vi "Periodic Tasks.vi"(8 "error in":errorcluster) -> ()   [LabVIEW 2012]
doc: "This VI runs in parallel to other tasks. It can contain as many user-defined periodic loops as you need. These can carry out PID or other sorts of timed response."
uses:
  <vilib>/Rock Robotics/WPI/Relay/WPI_RelayValue.ctl
  <vilib>/Rock Robotics/SystemInterfaces/Utilities/FPGA_UtilitiesLED Source.ctl
  <vilib>/Rock Robotics/SystemInterfaces/Utilities/FPGA_UtilitiesLED State.ctl
  Robot Global Data.vi
  <vilib>/Rock Robotics/WPI/Joystick/WPI_JoystickGetSetRefNum.vi
  <vilib>/Rock Robotics/WPI/RobotDrive/WPI_RobotDriveGetSetRefNum.vi
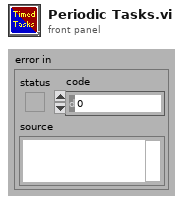
[diagram p1: front panel]
types:
  T1 = typedef "WPI_CompressorDevRef.ctl" = cluster{"DevStatus":errorcluster, "DigitalInputDevRef":T2, "RelayDevRef":T5}
  T2 = typedef "WPI_DigitalInputDevRef.ctl" = cluster{"DevStatus":errorcluster, "DIO Channel":T3, "Digital Module":T4}
  T3 = typedef "FPGA_DIOChannel.ctl" = enum8{"DIO 1", "DIO 2", "DIO 3", "DIO 4", "DIO 5", "DIO 6", "DIO 7", "DIO 8", "DIO 9", "DIO 10", "DIO 11", "DIO 12", "DIO 13", "DIO 14", "Invalid"}
  T4 = typedef "FPGA_TypedefDigitalModule.ctl" = enum16{"Digital Module 1", "Digital Module 2"}
  T5 = typedef "WPI_RelayDevRef.ctl" = cluster{"DevStatus":errorcluster, "Relay Channel":T6, "Digital Module":T4, "Relay Direction":T7}
  T6 = typedef "FPGA_DIORelayChannel.ctl" = enum8{"Relay 1", "Relay 2", "Relay 3", "Relay 4", "Relay 5", "Relay 6", "Relay 7", "Relay 8", "Invalid"}
  T7 = typedef "WPI_RelayDirection.ctl" = enum16{"Both directions", "Forward only", "Reverse only"}
  T8 = typedef "FPGA_UtilitiesLED State.ctl" = enum16{"Off", "On", "Toggle"}
  T9 = typedef "FPGA_UtilitiesLED Source.ctl" = enum16{"User LED", "FPGA LED"}
  T10 = typedef "WPI_RobotDriveDevRef.ctl" = cluster{"DevStatus":errorcluster, "Motors[]":T11[], "Square Inputs":bool, "Max Output":dbl, "Isochronous":bool}
  T11 = typedef "WPI_MotorControlDeviceRef.ctl" = cluster{"DeviceStatus":errorcluster, "Type":enum16{"PWM", "CAN"}, "PWM":cluster{"Digital Module":T4, "PWM Channel":T12, "DeadBand":T13}, "CAN":cluster{"Device Number":u8, "Control Mode":T14, "Semaphore":T15, "Max Vout":dbl}, "Invert":bool, "TransformRef":T16, "InvTransformRef":T16}
  T12 = typedef "FPGA_DIOPWMChannel.ctl" = enum8{"PWM 1", "PWM 2", "PWM 3", "PWM 4", "PWM 5", "PWM 6", "PWM 7", "PWM 8", "PWM 9", "PWM 10", "Invalid"}
  T13 = typedef "WPI_PWMDeadband.ctl" = cluster{"Name":string, "maxPositivePwm":i32, "minPositivePwm":i32, "centerPwm":i32, "maxNegativePwm":i32, "minNegativePwm":i32, "angularRange":u16}
  T14 = typedef "WPI_CANJaguar_ControlMode.ctl" = enum8{"Percent VBus", "Current", "Speed", "Position", "Voltage"}
  T15 = typedef "Semaphore RefNum" = refnum<k1>
  T16 = typedef "WPI_PWMTransform_ConPane.ctl" = refnum<vi>
  T17 = typedef "WPI_JoystickDevRef.ctl" = cluster{"Device":T18}
  T18 = typedef "WPI_JoystickDeviceEnum.ctl" = enum16{"USB 1", "USB 2", "USB 3", "USB 4", "Kinect 1", "Kinect 2"}
  T19 = cluster{"JoystickDevRef":T17, "RobotDriveDevRef":T10}
  T20 = typedef "WPI_RelayValue.ctl" = enum16{"Off", "On", "Forward", "Reverse"}
  T21 = typedef "WPI_JoystickButtonState.ctl" = cluster{"Button 1":bool, "Button 2":bool, "Button 3":bool, "Button 4":bool, "Button 5":bool, "Button 6":bool, "Button 7":bool, "Button 8":bool, "Button 9":bool, "Button 10":bool, "Button 11":bool, "Button 12":bool}
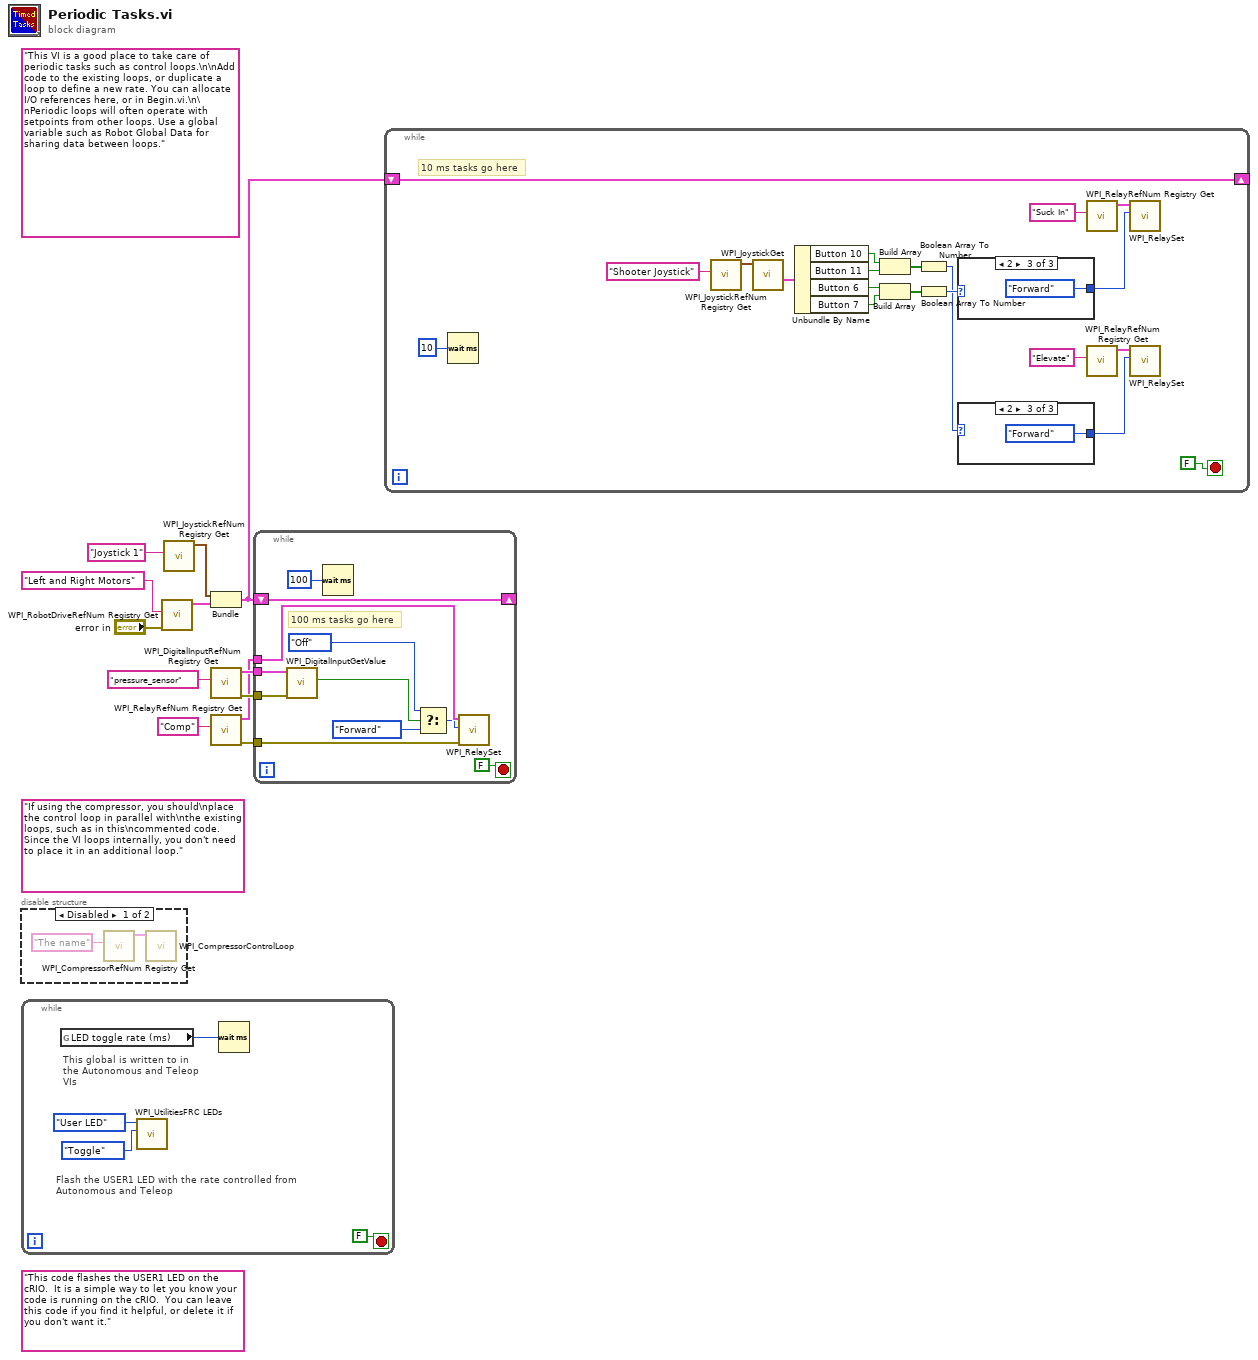
[diagram p0: block diagram]
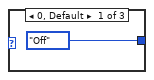
[diagram p3: hidden frame]
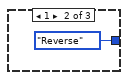
[diagram p4: hidden frame]
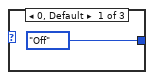
[diagram p5: hidden frame]
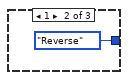
[diagram p6: hidden frame]
diagram:
  (unwired) "If using the compressor, you should\nplace the control loop in parallel with\nthe existing loops, such as in this\ncommented code. Since the VI loops internally, you don't need to place it in an additional loop."
  (unwired) "This code flashes the USER1 LED on the cRIO.  It is a simple way to let you know your code is running on the cRIO.  You can leave this code if you find it helpful, or delete it if you don't want it."
  (unwired) "This VI is a good place to take care of periodic tasks such as control loops.\n\nAdd code to the existing loops, or duplicate a loop to define a new rate. You can allocate I/O references here, or in Begin.vi.\n\nPeriodic loops will often operate with setpoints from other loops. Use a global variable such as Robot Global Data for sharing data between loops."
  n1 = disable-structure shown="Disabled" {
    frame Disabled {
      n2 = call <vilib>:"WPI_CompressorRefNum Registry Get.vi"("refnum name"="The name") -> ("CompressorDevRef"=w14:T1)  [unwired: 9 in, 1 out]
      n3 = call <vilib>:"WPI_CompressorControlLoop.vi"("CompressorDevRef"=w14) -> ()  [unwired: 11 in]
    }
    frame Enabled {
    }
  }
  n4 = while {
    stop <- FALSE stop-if-true
    # "This global is written to in the Autonomous and Teleop VIs"
    # "Flash the USER1 LED with the rate controlled from Autonomous and Teleop"
    n5 = global read "Robot Global Data.vi" "LED toggle rate (ms)"() -> (w15:u32)
    n6 = call <vilib>:"WPI_UtilitiesFRC LEDs.vi"("State"=FPGA_UtilitiesLED_State."Toggle", "LED Type"=FPGA_UtilitiesLED_Source."User LED") -> ()  [unwired: 1 in, 9 out]
    n7 = Wait (ms)(milliseconds to wait=w15) -> ()  [unwired: 1 out]
  }
  n8 = call <vilib>:"WPI_RobotDriveRefNum Registry Get.vi"("error in (no error)"="error in", "refnum name"="Left and Right Motors") -> ("RobotDriveDevRef"=w9:T10)  [unwired: 9 out]
  n9 = call <vilib>:"WPI_JoystickRefNum Registry Get.vi"("refnum name"="Joystick 1") -> ("JoystickDevRef"=w10:T17)  [unwired: 1 in, 9 out]
  n10 = Bundle("JoystickDevRef"=w10, "RobotDriveDevRef"=w9) -> (w8:T19)  [unwired: 1 out]
  n11 = call <vilib>:"WPI_DigitalInputRefNum Registry Get.vi"("refnum name"="pressure_sensor") -> ("error out"=w5:errorcluster, "DigitalInputDevRef"=w6:T2)  [unwired: 9 in]
  n12 = call <vilib>:"WPI_RelayRefNum Registry Get.vi"("refnum name"="Comp") -> ("error out"=w1:errorcluster, "RelayDevRef"=w2:T5)  [unwired: 9 in]
  n13 = while {
    shift-right: [w27] -> _
    shift-left: w8 -> [w27]
    tunnel: w6 -> [w26]
    tunnel: w5 -> [w25]
    tunnel: w2 -> [w24]
    tunnel: w1 -> [w23]
    stop <- FALSE stop-if-true
    # "100 ms tasks go here"
    n14 = call <vilib>:"WPI_DigitalInputGetValue.vi"("error in (no error)"=w25, "DigitalInputDevRef"=w26) -> ("Value"=w22:bool)  [unwired: 7 in, 2 out]
    n15 = Wait (ms)(milliseconds to wait=u32 100) -> ()  [unwired: 1 out]
    n16 = Select(t=WPI_RelayValue."Off" ("RelayValue"), s=w22, f=WPI_RelayValue."Forward" ("RelayValue")) -> (s? t:f=w19:T20)
    n17 = call <vilib>:"WPI_RelaySet.vi"("error in (no error)"=w23, "RelayValue"=w19, "RelayDevRef"=w24) -> ()  [unwired: 7 in, 2 out]
  }
  n18 = while {
    shift-right: [w47] -> _
    shift-left: w8 -> [w47]
    stop <- FALSE stop-if-true
    # "10 ms tasks go here"
    n19 = Wait (ms)(milliseconds to wait=u32 10) -> ()  [unwired: 1 out]
    n20 = call <vilib>:"WPI_JoystickRefNum Registry Get.vi"("refnum name"="Shooter Joystick") -> ("JoystickDevRef"=w31:T17)  [unwired: 1 in, 9 out]
    n21 = call <vilib>:"WPI_JoystickGet.vi"("JoystickDevRef"=w31) -> ("Buttons"=w32:T21)  [unwired: 1 in, 5 out]
    n22 = Unbundle By Name(w32) -> ("Button 10"=w41:bool, "Button 11"=w42:bool, "Button 6"=w33:bool, "Button 7"=w34:bool)
    n23 = Build Array(w41, w42) -> (w39:bool[])
    n24 = Build Array(w33, w34) -> (w35:bool[])
    n25 = Boolean Array To Number(Boolean array=w39) -> (number=w38:u32)
    n26 = Boolean Array To Number(Boolean array=w35) -> (number=w46:u32)
    n27 = case shown="2" w46 {
      tunnel: [WPI_RelayValue."Off" ("RelayValue") WPI_RelayValue."Reverse" ("RelayValue") WPI_RelayValue."Forward" ("RelayValue")] -> w44
      frame 0, Default {
      }
      frame 1 {
      }
      frame 2 {
      }
    }
    n28 = case shown="2" w38 {
      tunnel: [WPI_RelayValue."Off" ("RelayValue") WPI_RelayValue."Reverse" ("RelayValue") WPI_RelayValue."Forward" ("RelayValue")] -> w40
      frame 0, Default {
      }
      frame 1 {
      }
      frame 2 {
      }
    }
    n29 = call <vilib>:"WPI_RelayRefNum Registry Get.vi"("refnum name"="Suck In") -> ("RelayDevRef"=w43:T5)  [unwired: 9 in, 1 out]
    n30 = call <vilib>:"WPI_RelayRefNum Registry Get.vi"("refnum name"="Elevate") -> ("RelayDevRef"=w36:T5)  [unwired: 9 in, 1 out]
    n31 = call <vilib>:"WPI_RelaySet.vi"("RelayValue"=w44, "RelayDevRef"=w43) -> ()  [unwired: 8 in, 2 out]
    n32 = call <vilib>:"WPI_RelaySet.vi"("RelayValue"=w40, "RelayDevRef"=w36) -> ()  [unwired: 8 in, 2 out]
  }
